vi "f_MGCC_EnergyMgmt_CostSavings.vi"() -> ()   [LabVIEW 2016, in "MGCC_EnergyMgmt_dataIO.lvlib"]
uses:
  Lib/MGCC_EnergyMgmt_dataIO.lvlib
panel:
  out "Savings":dbl
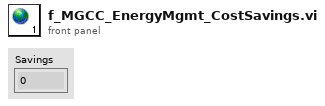
[diagram p1: front panel]
diagram:
